vi "XY Graph Delete Selected Plots Event.vi"(8 "Error In":errorcluster, 11 "XYGraph Ref":T1) -> (0 "Error Out":errorcluster, 1 "Message":string, 2 "Plot Names":string[](array[string]), 3 "Deleted Plot Indices":i32[](array[numeric]), 5 "Graph Caption":string)   [LabVIEW 2021, in "XY Graph Add-Ons.lvlib"]
uses:
  XY Graph Add-Ons.lvlib
  XY Graph Refnum.ctl
  Arrays/Arrays.lvlib
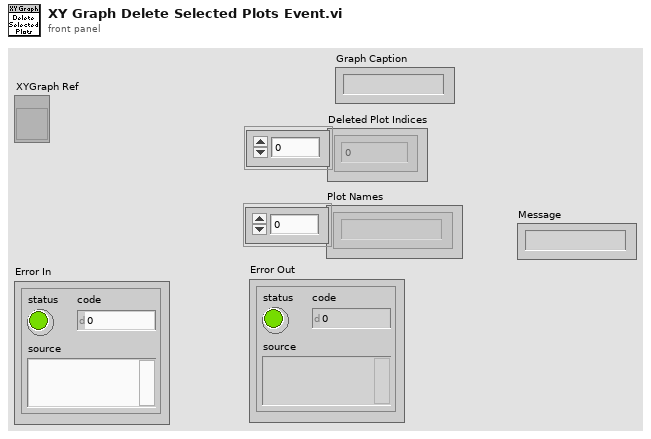
[diagram p1: front panel]
types:
  T1 = typedef "XY Graph Add-Ons.lvlib/XY Graph Refnum.ctl" = refnum<vi>
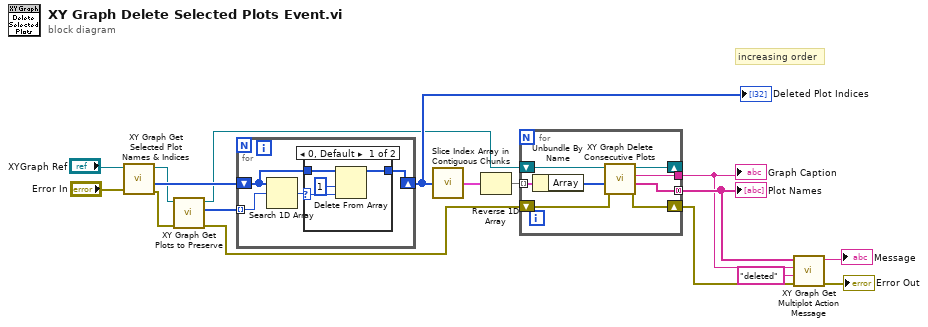
[diagram p0: block diagram]
diagram:
  # "increasing order"
  n1 = call "XY Graph Get Selected Plot Names & Indices.vi"("error in (no error)"="Error In", "XYGraph in"="XYGraph Ref") -> ("error out"=w8:errorcluster, "Selected Plots"=w15:i32[], "XYGraph out"=w11:T1)  [unwired: 5 in, 2 out]
  n2 = call "XY Graph Get Plots to Preserve.vi"("Error In"=w8, "XYGraph in"=w11) -> ("Error Out"=w7:errorcluster, "Preserved Plots"=w9:i32[], "XYGraph dup"=w10:T1)  [unwired: 6 in, 1 out]
  n3 = for {
    tunnel: w9 -> [w21] mode=indexing
    shift-right: [w18] -> w14
    shift-left: w15 -> [w19]
    n4 = Search 1D Array(1D array=w19, element=w21) -> (index of element=w20:i32)  [unwired: 1 in]
    n5 = case shown="0, Default" w20 {
      selector: w20 -> [w24 _]
      tunnel: w19 -> [w25 w26]
      tunnel: [w23 w26] -> w18
      frame 0, Default {
        n6 = Delete From Array(array=w25, length=1, index=w24) -> (array with subset deleted=w23:i32[])  [unwired: 1 out]
      }
      frame -1 {
      }
    }
  }
  "Deleted Plot Indices" <- w14
  n7 = call "Slice Index Array in Contiguous Chunks.vi"("Array in"=w14) -> ("Contiguous sub-Arrays"=w13:cluster{"Array":i32[]}[])  [unwired: 8 in]
  n8 = Reverse 1D Array(array=w13) -> (reversed array=w12:cluster{"Array":i32[]}[])
  n9 = for {
    tunnel: w12 -> [w34] mode=indexing
    shift-right: [w31] -> _
    shift-left: w10 -> [w32]
    tunnel: [w30] -> w5
    shift-right: [w28] -> w3
    shift-left: w7 -> [w29]
    tunnel: [w27] -> w6 mode=concatenating
    n10 = Unbundle By Name(w34) -> ("Array"=w33:i32[])
    n11 = call "XY Graph Delete Consecutive Plots.vi"("Error In"=w29, "Plot Indices"=w33, "XYGraph Ref"=w32) -> ("Error Out"=w28:errorcluster, "Plot Names"=w27:string[], "Graph Caption (or Label)"=w30:string, "XYGraph Ref"=w31:refnum<vi>)  [unwired: 5 in]
  }
  "Graph Caption" <- w5
  "Plot Names" <- w6
  n12 = call "XY Graph Get Multiplot Action Message.vi"("error in (no error)"=w3, "Graph Action"="deleted", "Graph Caption"=w5, "Plot Names"=w6) -> ("Error Out"=→"Error Out":errorcluster, "Multiplot Message"=→"Message":string)  [unwired: 6 in]
